vi "Wire All Terminals.vi"(6 "Variant in":variant, 7 "Shift Pressed?":bool, 8 "error in (no error)":errorcluster, 10 "QD Combo Box Ref":refnum<vi>, 11 "QD Launch VI Ref":refnum<vi>) -> (0 "error out":errorcluster, 4 "Variant out":variant)   [LabVIEW 2015]
doc: "Creates controls and indicators for all unwired inputs and outputs of the selected block diagram object(s). If 'shift' is also pressed, creates constants for all unwired inputs of the selected block diagram object(s).\n\nDefault Shortcut - [D]"
panel:
  in  "Undo Name":string="Create Inputs and/or Outputs"
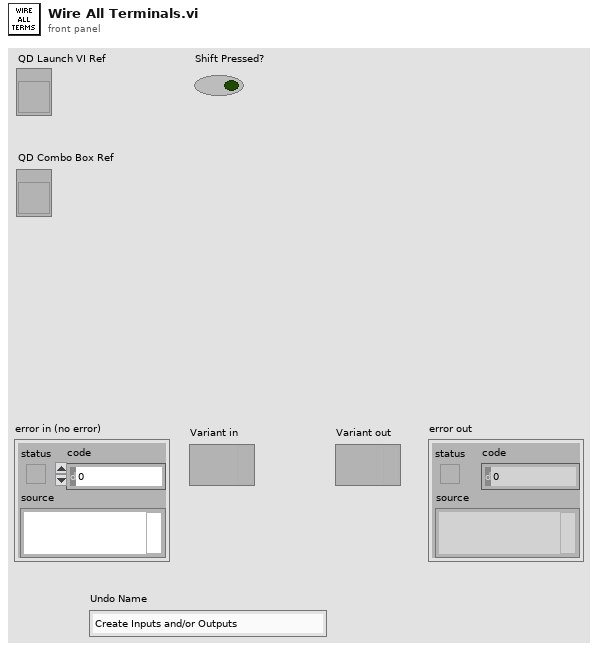
[diagram p1: front panel]
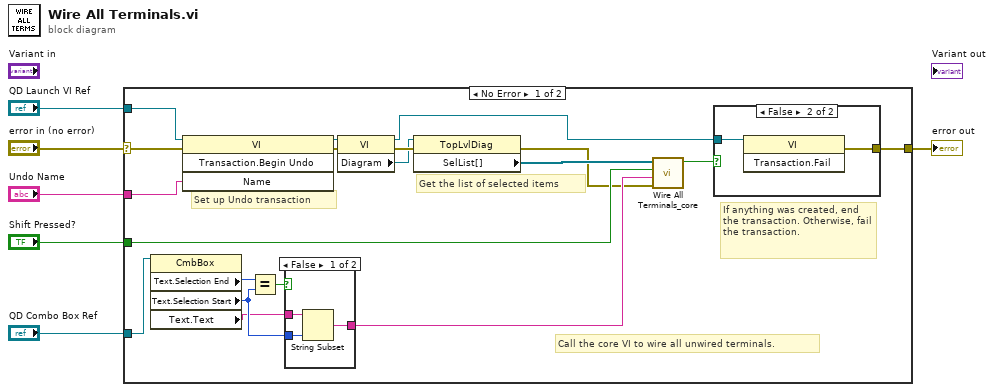
[diagram p0: block diagram]
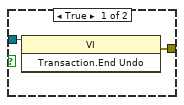
[diagram p3: hidden frame]
diagram:
  n1 = case shown="No Error" "error in (no error)" {
    selector: "error in (no error)" -> [w25 w34]
    tunnel: [w19 w34] -> w5
    tunnel: "Shift Pressed?" -> [w9 _]
    tunnel: "QD Combo Box Ref" -> [w14 _]
    tunnel: "QD Launch VI Ref" -> [w24 _]
    tunnel: "Undo Name" -> [w13 _]
    frame No Error {
      # "Call the core VI to wire all unwired terminals."
      # "If anything was created, end the transaction. Otherwise, fail the transaction."
      # "Get the list of selected items"
      # "Set up Undo transaction"
      n2 = property on="Property Node" class="CmbBox"(reference=w14) -> ("Text.Selection End"=w18:u32, "Text.Selection Start"=w16:u32, "Text.Text"=w15:string)  [unwired: 1 in, 2 out]
      n3 = invoke class="VI" method="Transaction.Begin Undo"(reference=w24, error in=w25, "Name"=w13) -> (reference out=w20:refnum<vi>, error out=w21:errorcluster)  [unwired: 1 in, 2 out]
      n4 = Equal?(x=w18, y=w16) -> (x = y?=w17:bool)
      n5 = case shown="False" w17 {
        tunnel: [w28 w29] -> w11
        tunnel: w16 -> [w27 _]
        tunnel: w15 -> [w26 w29]
        frame False {
          n6 = String Subset(string=w26, length (rest)=w27) -> (substring=w28:string)  [unwired: 1 out]
        }
        frame True {
        }
      }
      n7 = property class="VI"(reference=w20, error in=w21) -> (reference out=w12:refnum<vi>, error out=w23:errorcluster, "Diagram"=w22:refnum<vi>)
      n8 = property class="TopLvlDiag"(reference=w22, error in=w23) -> (error out=w7:errorcluster, "SelList[]"=w10:refnum<vi>[])  [unwired: 1 out]
      n9 = call <vilib>:"Wire All Terminals_core.vi"("error in (no error)"=w7, "User string"=w11, "Create constants?"=w9, "SelList[]"=w10) -> ("changes made?"=w8:bool)  [unwired: 6 in, 1 out]
      n10 = case shown="False" w8 {
        tunnel: w12 -> [w30 w32]
        tunnel: [w31 w33] -> w19
        frame True {
          n11 = invoke class="VI" method="Transaction.End Undo"(reference=w30) -> (error out=w31:errorcluster)  [unwired: 2 in, 2 out]
        }
        frame False {
          n12 = invoke class="VI" method="Transaction.Fail"(reference=w32) -> (error out=w33:errorcluster)  [unwired: 2 in, 2 out]
        }
      }
    }
    frame Error {
    }
  }
  "error out" <- w5
